vi "OSF Create Wiki.vi"(6 "content":string, 7 "OSF API URL":string="https://api.osf.io/v2/", 8 "error in":errorcluster, 9 "Wiki name":string, 10 "Parent  ID":string, 11 "client handle":T2) -> (0 "error out":errorcluster, 1 "Wiki ID":string, 2 "Responce body":string, 3 "client handle out":T2)   [LabVIEW 2020]
uses:
  <vilib>/httpClient/ClientHandle.ctl
  55103850-15ef-4a18-9388-7b0eadcdd449.vi
  <vilib>/JDP Science/JSONtext/Variant to JSON Text.vi
  <vilib>/httpClient/POSTBuffer.vi
  <vilib>/JDP Science/JSONtext/LVClass Serializer/JSONtext LVClass Serializer.lvclass
  <vilib>/httpClient/LabVIEWHTTPClient.lvlib
panel:
  in  "OSF Wiki":T1={"data"={"type"="wikis", "attributes"={"name"="", "content"=""}}}
  out "Puject  JSON":string
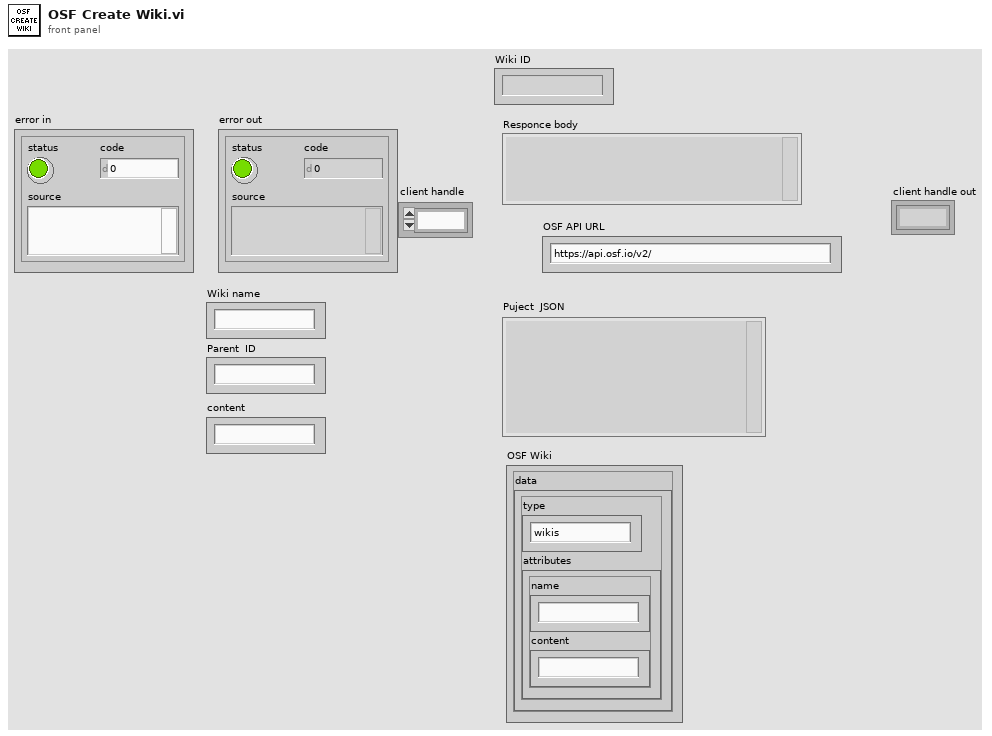
[diagram p1: front panel]
types:
  T1 = cluster{"data":cluster{"type":string, "attributes":cluster{"name":string, "content":string}}}
  T2 = typedef "LabVIEWHTTPClient.lvlib/ClientHandle.ctl" = refnum<k1>
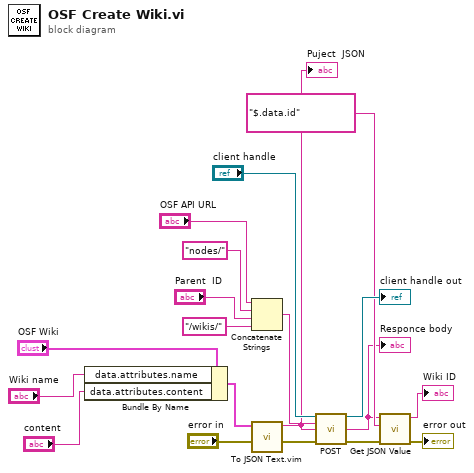
[diagram p0: block diagram]
diagram:
  n1 = Bundle By Name(cluster="OSF Wiki", "data.attributes.name"="Wiki name", "data.attributes.content"="content") -> (w19:T1)
  n2 = Concatenate Strings("OSF API URL", "nodes/", "Parent  ID", "/wikis/" ("string")) -> (w10:string)
  n3 = call "To JSON Text.vim"("error in (no error)"="error in", "Anything"=w19) -> ("error out"=w9:errorcluster, "<JSON>"=w7:string)  [unwired: 8 in]
  "Puject  JSON" <- w7
  n4 = call-poly <vilib>:"POST.vi"("client handle"="client handle", "url"=w10, "buffer"=w7, "error in (no error)"=w9) -> ("client handle out"=→"client handle out":T2, "body"=w2:string, "error out"=w4:errorcluster)  [unwired: 8 in, 1 out]
  "Responce body" <- w2
  n5 = call "Get JSON Value.vi"("error in"=w4, "$Path or Item Name"="$.data.id", "JSON in"=w2) -> ("error out"=→"error out":errorcluster, "Value"=→"Wiki ID":string)  [unwired: 5 in, 2 out]
